vi "Register.vi"(8 "error in (no error)":errorcluster, 11 "logger in":refnum<class "Logger.lvclass">) -> (0 "error out":errorcluster)   [LabVIEW 2024, in "Logging.lvlib" / "Registry.lvlib"]
uses:
  Registry.lvlib
  Logger/Logger.lvclass
  Registry Actions.ctl
panel:
  # "Connector Pane"
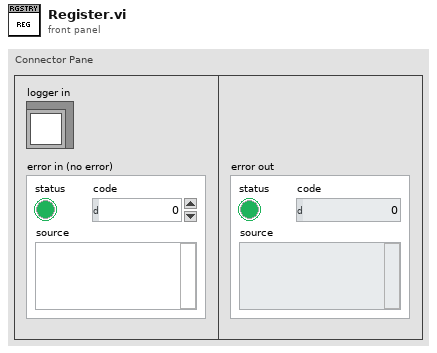
[diagram p1: front panel]
types:
  T1 = typedef "Logging.lvlib/Registry.lvlib/Registry Actions.ctl" = enum16{"Register", "Log", "List", "Unregister", "Unregister All"}
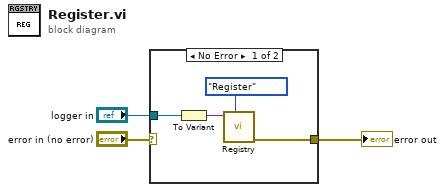
[diagram p0: block diagram]
diagram:
  n1 = case shown="No Error" "error in (no error)" {
    selector: "error in (no error)" -> [_ w8]
    tunnel: "logger in" -> [w6 _]
    tunnel: [w4 w8] -> w2
    frame No Error {
      n2 = To Variant(anything=w6) -> (Variant=w5:variant)
      n3 = call "Registry.vi"("action"=Registry_Actions."Register", "data in"=w5) -> ("error out"=w4:errorcluster)  [unwired: 8 in, 1 out]
    }
    frame Error {
    }
  }
  "error out" <- w2
